vi "10_DiDt_OFF.vi"(0 "file path (IN)":path, 1 "ICE":dbl, 5 "Project #":string, 7 "Request #":string, 9 "TEST #":string, 11 "error in (no error)":errorcluster) -> (4 "file path (OUT)":path, 6 "Di/Dt (A/us)":dbl, 8 "DONE Di/Dt OFF":bool, 10 "OFF Region":waveform(dbl)[](graph) caption="DiDtOff (A/us)", 13 "Di (A)":dbl, 14 "Dt (ns)":dbl, 15 "error out":errorcluster)   [LabVIEW 2020]
uses:
  <vilib>/Waveform/WDTOps.llb/WDT Waveform Duration DBL.vi
  <vilib>/Waveform/WDTOps.llb/WDT Get Waveform Subset DBL.vi
  <vilib>/measure/mascope.llb/Transition Measurements 1 chan.vi
  <vilib>/measure/NI_MAPro.lvlib
panel:
  in  "Decision ?":bool
  out "Cursor b : Channel 1":dbl
  out "Cursor a : Channel 1":dbl
  in  "Cursor b : Channel 1 \nfall edge number":i32=1 min=1
  in  "Cursor b : Channel 1 \nfall edge tolerance":dbl=0.1
  in  "Cursor a : Channel 1 \nfall edge tolerance":dbl=0.1
  in  "Cursor a : Channel 1 \nfall edge number":i32=1 min=1
  out "Dt (us)":dbl
  out "50% Ice":dbl
  out "90% Ice":dbl
  out "measurement info (CH1 Cursor a)":T1 {"ref levels"."ref units" items=["absolute", "relative"]; "ref levels"."high ref level" format="%.2p"; "ref levels"."low ref level" format="%.2p"; "ref levels"."mid ref level" format="%.2p"; "end time" format="%.6e"; "start time" format="%.6e"}
  out "measurement info (CH1 Cursor b)":T1 {"ref levels"."ref units" items=["absolute", "relative"]; "ref levels"."high ref level" format="%.2p"; "ref levels"."low ref level" format="%.2p"; "ref levels"."mid ref level" format="%.2p"; "end time" format="%.6e"; "start time" format="%.6e"}
  in  "reference  levels (CH1 2nd Cursor)":T2={"high ref level"=90.0, "mid ref level"=50.0, "low ref level"=10.0, "ref units"=1} {"ref units" items=["absolute", "percent"]; "high ref level" format="%0.2f"; "low ref level" format="%0.2f"; "mid ref level" format="%0.2f"}
  in  "reference  levels (CH1 1st Cursor)":T2={"high ref level"=90.0, "mid ref level"=50.0, "low ref level"=10.0, "ref units"=1} {"ref units" items=["absolute", "percent"]; "high ref level" format="%0.2f"; "low ref level" format="%0.2f"; "mid ref level" format="%0.2f"}
  out "Waveform Graph":waveform(dbl)[](graph)
  # "From 90% to 50% of Nominal Current"
  # "Default = 1"
  # "Default = 1"
  # "Default = 0.1"
  # "Default = 0.1"
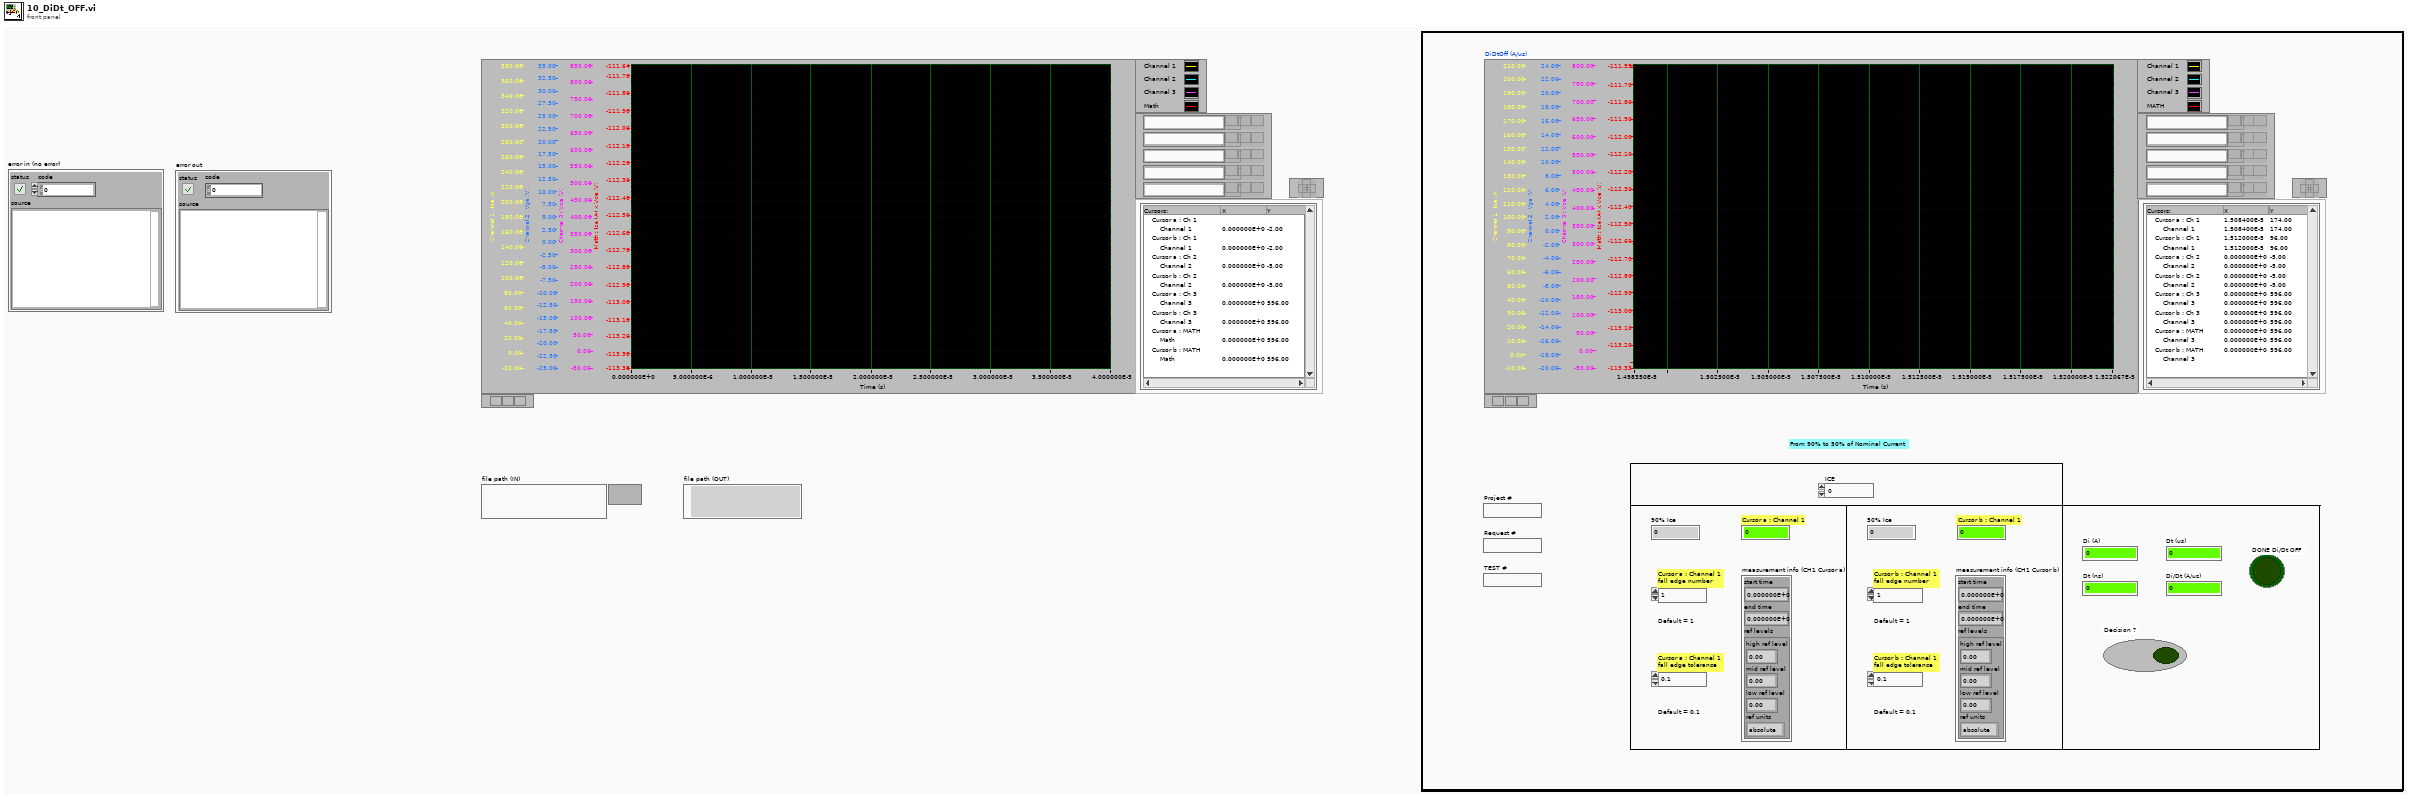
[diagram p1: front panel]
types:
  T1 = cluster{"start time":dbl, "end time":dbl, "ref levels":cluster{"high ref level":dbl, "mid ref level":dbl, "low ref level":dbl, "ref units":u16}}
  T2 = cluster{"high ref level":dbl, "mid ref level":dbl, "low ref level":dbl, "ref units":u16}
  T3 = enum32{"Invalid", "Standard", "Closed", "Hidden", "Minimized", "Maximized"}
  T4 = typedef "imagedata.ctl" = cluster{"image type":i32, "image depth":i32, "image":u8[], "mask":u8[], "colors":u32[], "Rectangle":cluster{"left":i16, "top":i16, "right":i16, "bottom":i16}}
diagram:
  w12 = 0.0 ("Di (A)")
  w13 = errorcluster {"status"=FALSE, "code"=0, "source"=""} ("error out")
  w11 = FALSE ("DONE Tdon")
  w14 = waveform(dbl)[] [] ("Waveform Graph")
  n1 = disable-structure shown="Disabled" {
    frame Disabled {
      n2 = control-ref of="This VI"() -> (w15:refnum<vi>)
      n3 = control-ref of="This VI"() -> (w16:refnum<vi>)
      n4 = invoke class="VI" method="FP.Close"(reference=w15) -> ()  [unwired: 2 in, 3 out]
      n5 = invoke class="VI" method="FP.Open"(reference=w16, "Activate"=TRUE ("Activate?"), "State"=T3."Maximized") -> (error in=w19:errorcluster, error out=w17:errorcluster)  [unwired: 1 in, 4 out]
      n6 = property class="VI"(reference=w16, error in=w17, "Front Panel.Closeable"=TRUE ("Front Panel Window:Closeable")) -> ()  [unwired: 2 out]
    }
    frame Enabled {
    }
  }
  n7 = local write "Cursor a : Channel 1 \nfall edge tolerance"(0.1 ("Cursor a : Channel 1 \nfall edge tolerance")) -> ()
  n8 = local write "Cursor a : Channel 1 \nfall edge number"(1 ("Cursor a : Channel 1 \nfall edge number")) -> ()
  n9 = local write "Cursor b : Channel 1 \nfall edge number"(1 ("Cursor b : Channel 1 \nfall edge number")) -> ()
  n10 = local write "Cursor b : Channel 1 \nfall edge tolerance"(0.1 ("Cursor b : Channel 1 \nfall edge tolerance")) -> ()
  n11 = local write "Cursor a : Channel 1"(w12) -> ()
  n12 = local write "Cursor b : Channel 1"(w12) -> ()
  n13 = local write "Di (A)"(w12) -> ()
  n14 = local write "Dt (ns)"(w12) -> ()
  n15 = local write "Dt (us)"(w12) -> ()
  n16 = local write "Di/Dt (A/us)"(w12) -> ()
  n17 = local write "error out"(w13) -> ()
  n18 = local write "error in (no error)"(w13) -> ()
  n19 = local write "DONE Di/Dt OFF"(w11) -> ()
  n20 = local write "Waveform Graph"(w14) -> ()
  n21 = local write "OFF Region"(w14) -> ()
  n22 = local write "Decision ?"(w11) -> ()
  n23 = flat-sequence {
    tunnel: [w22] -> w6
    tunnel: ["file path (IN)"] -> w5
    tunnel: [w33] -> w10
    tunnel: [w32] -> w8
    tunnel: w6 -> [w31]
    tunnel: w5 -> [w30]
    tunnel: w10 -> [w265]
    tunnel: [w264] -> w9
    tunnel: w8 -> [w264]
    tunnel: [w263] -> w7
    tunnel: w9 -> [w279]
    tunnel: w7 -> [w278]
    frame #0 {
      n24 = control-ref of="This VI"() -> (w27:refnum<vi>)
      n25 = invoke class="VI" method="FP.Open"(reference=w27, error in="error in (no error)", "Activate"=TRUE ("Activate?"), "State"=T3."Maximized") -> (error out=w28:errorcluster)  [unwired: 1 in, 4 out]
      n26 = property class="VI"(reference=w27, error in=w28, "Front Panel.Closeable"=TRUE ("Front Panel Window:Closeable")) -> (error out=w22:errorcluster)  [unwired: 1 out]
    }
    frame #1 {
      n27 = while {
        tunnel: [w37] -> w32
        shift-right: [w38] -> w33
        shift-left: w31 -> [w36]
        tunnel: w30 -> [w35]
        stop <- w40 stop-if-true
        n28 = flat-sequence {
          tunnel: [w71] -> w59
          tunnel: w36 -> [w71]
          tunnel: w35 -> [w66]
          tunnel: [w66] -> w34
          tunnel: w59 -> [w164]
          tunnel: [w87] -> w58
          tunnel: [w86] -> w57
          tunnel: [w76] -> w56
          tunnel: w34 -> [w158]
          tunnel: w58 -> [w193]
          tunnel: w57 -> [w207]
          tunnel: [w187] -> w55
          tunnel: w56 -> [w200]
          tunnel: [w200] -> w54
          tunnel: [w178] -> w53
          tunnel: [w177] -> w52
          tunnel: [w186] -> w51
          tunnel: [w185] -> w50
          tunnel: w55 -> [w234]
          tunnel: [w235] -> w49
          tunnel: w54 -> [w238]
          tunnel: [w238] -> w48
          tunnel: w53 -> [w237]
          tunnel: [w237] -> w47
          tunnel: w52 -> [w236]
          tunnel: [w236] -> w46
          tunnel: w51 -> [w228]
          tunnel: [w228] -> w45
          tunnel: w50 -> [w229]
          tunnel: [w229] -> w44
          tunnel: w49 -> [w239]
          tunnel: w48 -> [w252]
          tunnel: [w252] -> w43
          tunnel: w47 -> [w246]
          tunnel: w46 -> [w247]
          tunnel: w45 -> [w245]
          tunnel: w44 -> [w244]
          tunnel: [w239] -> w42
          tunnel: w43 -> [w257]
          tunnel: w42 -> [w259]
          tunnel: [w258] -> w41
          tunnel: [w257] -> w37
          frame #0 {
            w69 = 0.0 ("Di (A)")
            w70 = FALSE ("DONE Tdon")
            w68 = waveform(dbl)[] [] ("Waveform Graph")
            n29 = Wait (ms)(milliseconds to wait=u32 200) -> ()  [unwired: 1 out]
            n30 = local write "Cursor a : Channel 1"(w69) -> ()
            n31 = local write "Cursor b : Channel 1"(w69) -> ()
            n32 = local write "Di/Dt (A/us)"(w69) -> ()
            n33 = local write "Dt (us)"(w69) -> ()
            n34 = local write "Di (A)"(w69) -> ()
            n35 = local write "Dt (ns)"(w69) -> ()
            n36 = local write "DONE Di/Dt OFF"(w70) -> ()
            n37 = local write "Waveform Graph"(w68) -> ()
            n38 = local write "OFF Region"(w68) -> ()
            n39 = local write "Decision ?"(w70) -> ()
          }
          frame #1 {
            w72 = 0.0 ("start samples/time")
            w139 = u16 1 items=["Samples", "Relative Time"] ("start/duration format")
            w150 = u16 1 items=["Samples", "Relative Time"] ("start/duration format")
            w151 = u16 1 items=["Samples", "Relative Time"] ("start/duration format")
            # "Channel 1"
            # "Channel 3"
            # "Channel 2"
            # "dt"
            # "Ch2"
            # "Ch1"
            n40 = call "3_ReadDatatoWaveform.vi"("error in (no error)"=w164, "file path (IN)"=w158) -> ("error out"=w132:errorcluster, "Waveform Graph"=→"Waveform Graph":waveform(dbl)[], "file path (OUT)"=w76:path, "dt"=w159:dbl, "Ch 2 Data"=w156:dbl[], "Ch 3 Data"=w160:dbl[], "Ch 1 Data"=w157:dbl[])  [unwired: 3 in]
            n41 = To Time Stamp(1:0.0 ("number")) -> (0:w161:timestamp)
            n42 = disable-structure shown="Enabled" {
              disable-tunnel: w161 -> [w168 _]
              disable-tunnel: w159 -> [w167 _]
              disable-tunnel: w157 -> [w166 _]
              disable-tunnel: [w165 _] -> w138
              frame Enabled {
                # "Channel 1"
                n43 = Bundle By Name("Y"=w166, "dt"=w167, "t0"=w168) -> (w165:waveform(dbl))  [unwired: 1 in]
              }
              frame Disabled {
              }
            }
            n44 = disable-structure shown="Enabled" {
              disable-tunnel: w161 -> [w172 _]
              disable-tunnel: w159 -> [w171 _]
              disable-tunnel: w156 -> [w170 _]
              disable-tunnel: [w169 _] -> w137
              frame Enabled {
                # "Channel 2"
                n45 = Bundle By Name("Y"=w170, "dt"=w171, "t0"=w172) -> (w169:waveform(dbl))  [unwired: 1 in]
              }
              frame Disabled {
              }
            }
            n46 = disable-structure shown="Enabled" {
              disable-tunnel: w161 -> [w176 _]
              disable-tunnel: w159 -> [w175 _]
              disable-tunnel: w160 -> [w174 _]
              disable-tunnel: [w173 _] -> w136
              frame Enabled {
                # "Channel 3"
                n47 = Bundle By Name("Y"=w174, "dt"=w175, "t0"=w176) -> (w173:waveform(dbl))  [unwired: 1 in]
              }
              frame Disabled {
              }
            }
            n48 = call-poly <vilib>:"Waveform Duration.vi"("error in (no error)"=w132, "waveform in"=w136) -> ("error out"=w144:errorcluster, "duration"=w141:dbl, "waveform out"=w143:waveform(dbl))  [unwired: 7 in]
            n49 = call-poly <vilib>:"Waveform Duration.vi"("error in (no error)"=w132, "waveform in"=w137) -> ("error out"=w145:errorcluster, "duration"=w148:dbl, "waveform out"=w146:waveform(dbl))  [unwired: 7 in]
            n50 = call-poly <vilib>:"Waveform Duration.vi"("error in (no error)"=w132, "waveform in"=w138) -> ("error out"=w155:errorcluster, "duration"=w152:dbl, "waveform out"=w154:waveform(dbl))  [unwired: 7 in]
            n51 = Divide(x=w141, y=2.0) -> (x/y=w140:dbl)
            n52 = Divide(x=w148, y=2.0) -> (x/y=w149:dbl)
            n53 = Divide(x=w152, y=2.0) -> (x/y=w133:dbl)
            n54 = call-poly <vilib>:"Get Waveform Subset.vi"("start/duration format"=w139, "error in (no error)"=w144, "duration"=w140, "start samples/time"=w72, "waveform in"=w143) -> ("error out"=w129:errorcluster, "waveform out"=w135:waveform(dbl))  [unwired: 1 in, 2 out]
            n55 = call-poly <vilib>:"Get Waveform Subset.vi"("start/duration format"=w150, "error in (no error)"=w145, "duration"=w149, "start samples/time"=w72, "waveform in"=w146) -> ("error out"=w130:errorcluster, "waveform out"=w88:waveform(dbl))  [unwired: 1 in, 2 out]
            n56 = call-poly <vilib>:"Get Waveform Subset.vi"("start/duration format"=w151, "error in (no error)"=w155, "duration"=w133, "start samples/time"=w72, "waveform in"=w154) -> ("error out"=w131:errorcluster, "waveform out"=w87:waveform(dbl))  [unwired: 1 in, 2 out]
            n57 = Build Array(w87, w88, w135) -> (→"OFF Region":waveform(dbl)[])
            n58 = Merge Errors(w131, w130, w129) -> (w84:errorcluster)
            n59 = property on="OFF Region" class="WFGraph (strict)"(error in=w84) -> (error out=w83:errorcluster, "Width"=w82:u32)  [unwired: 1 in, 1 out]
            n60 = property on="OFF Region" class="WFGraph (strict)"(error in=w83, "Caption.Justify"=enum16{"Left", "Center", "Right"}."Left" ("Caption.Justification"), "Caption.Width"=w82, "Caption.FontBold"=TRUE ("Caption.Font:Bold"), "Caption.FontColor"=u32 16860 ("Caption.Font:Color"), "Caption.FontSize"=u32 24 ("Caption.Font:Size"), "Caption.Text"="DiDtOff (A/us)") -> (error out=w78:errorcluster)  [unwired: 1 in, 1 out]
            n61 = property on="OFF Region" class="WFGraph (strict)"(error in=w78, "XScale.Offset"=w72) -> (error out=w112:errorcluster)  [unwired: 1 in, 1 out]
            n62 = property on="OFF Region" class="WFGraph (strict)"(error in=w112, "Active Cursor"=u32 0, "Cursor.Cursor X"=0.0 ("Cursor.Cursor Position:Cursor X"), "Cursor.Cursor Y"=0.0 ("Cursor.Cursor Position:Cursor Y"), "Cursor.Visible"=FALSE) -> (error out=w111:errorcluster)  [unwired: 1 in, 1 out]
            n63 = property on="OFF Region" class="WFGraph (strict)"(error in=w111, "Active Cursor"=u32 1, "Cursor.Cursor X"=0.0 ("Cursor.Cursor Position:Cursor X"), "Cursor.Cursor Y"=0.0 ("Cursor.Cursor Position:Cursor Y"), "Cursor.Visible"=FALSE) -> (error out=w110:errorcluster)  [unwired: 1 in, 1 out]
            n64 = property on="OFF Region" class="WFGraph (strict)"(error in=w110, "Active Cursor"=u32 2, "Cursor.Cursor X"=0.0 ("Cursor.Cursor Position:Cursor X"), "Cursor.Cursor Y"=0.0 ("Cursor.Cursor Position:Cursor Y"), "Cursor.Visible"=FALSE) -> (error out=w109:errorcluster)  [unwired: 1 in, 1 out]
            n65 = property on="OFF Region" class="WFGraph (strict)"(error in=w109, "Active Cursor"=u32 3, "Cursor.Cursor X"=0.0 ("Cursor.Cursor Position:Cursor X"), "Cursor.Cursor Y"=0.0 ("Cursor.Cursor Position:Cursor Y"), "Cursor.Visible"=FALSE) -> (error out=w92:errorcluster)  [unwired: 1 in, 1 out]
            n66 = property on="OFF Region" class="WFGraph (strict)"(error in=w92, "Active Cursor"=u32 4, "Cursor.Cursor X"=0.0 ("Cursor.Cursor Position:Cursor X"), "Cursor.Cursor Y"=0.0 ("Cursor.Cursor Position:Cursor Y"), "Cursor.Visible"=FALSE) -> (error out=w91:errorcluster)  [unwired: 1 in, 1 out]
            n67 = property on="OFF Region" class="WFGraph (strict)"(error in=w91, "Active Cursor"=u32 5, "Cursor.Cursor X"=0.0 ("Cursor.Cursor Position:Cursor X"), "Cursor.Cursor Y"=0.0 ("Cursor.Cursor Position:Cursor Y"), "Cursor.Visible"=FALSE) -> (error out=w90:errorcluster)  [unwired: 1 in, 1 out]
            n68 = property on="OFF Region" class="WFGraph (strict)"(error in=w90, "Active Cursor"=u32 6, "Cursor.Cursor X"=0.0 ("Cursor.Cursor Position:Cursor X"), "Cursor.Cursor Y"=0.0 ("Cursor.Cursor Position:Cursor Y"), "Cursor.Visible"=FALSE) -> (error out=w89:errorcluster)  [unwired: 1 in, 1 out]
            n69 = property on="OFF Region" class="WFGraph (strict)"(error in=w89, "Active Cursor"=u32 7, "Cursor.Cursor X"=0.0 ("Cursor.Cursor Position:Cursor X"), "Cursor.Cursor Y"=0.0 ("Cursor.Cursor Position:Cursor Y"), "Cursor.Visible"=FALSE) -> (error out=w86:errorcluster)  [unwired: 1 in, 1 out]
            n70 = call <vilib>:"Beep.vi"("use system alert? (T)"=FALSE, "duration (msec)"=u32 200, "frequency (Hz)"=u32 2000) -> ()  [unwired: 9 in]
          }
          frame #2 {
            w220 = u16 0 items=["falling", "rising"] ("polarity (rising)")
            w221 = u16 0 items=["falling", "rising"] ("polarity (rising)")
            # "XPOS"
            # "YPOS"
            # "Cursor a : Channel 1"
            # "Cursor b : Channel 1"
            # "Cursor b : Channel 1"
            # "Cursor a : Channel 1"
            # "Cursor b : Channel 1"
            # "Cursor a : Channel 1"
            # "Cursor b : Channel 1"
            # "Cursor a : Channel 1"
            # "End Time 1st Cursor"
            # "End Time 2nd Cursor"
            # "1st PARAMETER : 90% Ice"
            # "Channel 1"
            # "2nd PARAMETER : 50% Ice"
            # "Channel 1"
            n71 = Divide(x=90.0, y=100.0) -> (x/y=w227:dbl)
            n72 = Multiply(x=w227, y="ICE") -> (x*y=w195:dbl)
            "90% Ice" <- w195
            n73 = Add(x=w195, y="Cursor a : Channel 1 \nfall edge tolerance") -> (x+y=w213:dbl)
            n74 = Subtract(x=w195, y="Cursor a : Channel 1 \nfall edge tolerance") -> (x-y=w212:dbl)
            n75 = Bundle By Name(cluster="reference  levels (CH1 1st Cursor)", "high ref level"=w213, "mid ref level"=w195, "low ref level"=w212, "ref units"=u16 0) -> (w209:T2)
            n76 = call-poly <vilib>:"Transition Measurements.vi"("edge number (1)"="Cursor a : Channel 1 \nfall edge number", "error in (no error)"=w207, "reference levels"=w209, "polarity (rising)"=w221, "signal in"=w193) -> ("error out"=w204:errorcluster, "measurement info"=w208:T1)  [unwired: 1 in, 4 out]
            "measurement info (CH1 Cursor a)" <- w208
            n77 = Unbundle By Name(w208) -> ("end time"=w185:dbl)
            n78 = property on="OFF Region" class="WFGraph (strict)"(error in=w204, "Active Cursor"=u32 0, "Cursor.Cursor X"=w185, "Cursor.Visible"=TRUE, "Cursor.Cursor Name Visible"=TRUE) -> (error out=w192:errorcluster)  [unwired: 1 in, 1 out]
            n79 = property on="OFF Region" class="WFGraph (strict)"(error in=w192, "Active Cursor"=u32 0) -> (error out=w190:errorcluster, "Cursor.Cursor Y"=w178:dbl)  [unwired: 1 in, 1 out]
            "Cursor a : Channel 1" <- w178
            n80 = Divide(x=50.0, y=100.0) -> (x/y=w224:dbl)
            n81 = Multiply(x=w224, y="ICE") -> (x*y=w196:dbl)
            "50% Ice" <- w196
            n82 = Add(x=w196, y="Cursor b : Channel 1 \nfall edge tolerance") -> (x+y=w219:dbl)
            n83 = Subtract(x=w196, y="Cursor b : Channel 1 \nfall edge tolerance") -> (x-y=w218:dbl)
            n84 = Bundle By Name(cluster="reference  levels (CH1 2nd Cursor)", "high ref level"=w219, "mid ref level"=w196, "low ref level"=w218, "ref units"=u16 0) -> (w215:T2)
            n85 = call-poly <vilib>:"Transition Measurements.vi"("edge number (1)"="Cursor b : Channel 1 \nfall edge number", "error in (no error)"=w190, "reference levels"=w215, "polarity (rising)"=w220, "signal in"=w193) -> ("error out"=w201:errorcluster, "measurement info"=w214:T1)  [unwired: 1 in, 4 out]
            "measurement info (CH1 Cursor b)" <- w214
            n86 = Unbundle By Name(w214) -> ("end time"=w186:dbl)
            n87 = property on="OFF Region" class="WFGraph (strict)"(error in=w201, "Active Cursor"=u32 1, "Cursor.Cursor X"=w186, "Cursor.Visible"=TRUE, "Cursor.Cursor Name Visible"=TRUE) -> (error out=w188:errorcluster)  [unwired: 1 in, 1 out]
            n88 = call <vilib>:"Beep.vi"("use system alert? (T)"=FALSE, "duration (msec)"=u32 200, "frequency (Hz)"=u32 2000) -> ()  [unwired: 9 in]
            n89 = property on="OFF Region" class="WFGraph (strict)"(error in=w188, "Active Cursor"=u32 1) -> (error out=w187:errorcluster, "Cursor.Cursor Y"=w177:dbl)  [unwired: 1 in, 1 out]
            "Cursor b : Channel 1" <- w177
          }
          frame #3 {
            # "2nd Cursor"
            # "1st Cursor"
            n90 = Subtract(x=w229, y=1e-07) -> (x-y=w230:dbl)
            n91 = Add(x=w228, y=1e-07) -> (x+y=w231:dbl)
            n92 = property on="OFF Region" class="WFGraph (strict)"(error in=w234, "XScale.Minimum"=w230, "XScale.Maximum"=w231) -> (error out=w235:errorcluster)  [unwired: 1 in, 1 out]
          }
          frame #4 {
            # "us"
            # "ns"
            n93 = Subtract(x=w247, y=w246) -> (x-y=w242:dbl)
            n94 = Subtract(x=w245, y=w244) -> (x-y=w243:dbl)
            n95 = Absolute Value(x=w242) -> (abs(x)=w241:dbl)
            "Di (A)" <- w241
            n96 = Absolute Value(x=w243) -> (abs(x)=w240:dbl)
            n97 = Multiply(x=w240, y=1000000000.0) -> (x*y=→"Dt (ns)":dbl)
            n98 = Multiply(x=w240, y=1000000.0) -> (x*y=w249:dbl)
            "Dt (us)" <- w249
            n99 = Divide(x=w241, y=w249) -> (x/y=→"Di/Dt (A/us)":dbl)
            n100 = call <vilib>:"Beep.vi"("use system alert? (T)"=FALSE, "duration (msec)"=u32 200, "frequency (Hz)"=u32 2000) -> ()  [unwired: 9 in]
          }
          frame #5 {
            n101 = while {
              shift-right: [w260] -> w258
              shift-left: w259 -> [w260]
              stop <- "Decision ?" stop-if-true
              n102 = Wait (ms)(milliseconds to wait=u32 100) -> ()  [unwired: 1 out]
            }
          }
        }
        n103 = while {
          tunnel: [w61] -> w40
          shift-right: [w64] -> w38
          shift-left: w41 -> [w65]
          stop <- w63 stop-if-true
          n104 = Wait (ms)(milliseconds to wait=u32 100) -> ()  [unwired: 1 out]
          n105 = call "Display Message to User"("error in (no error)"=w65) -> ("error out"=w64:errorcluster, "NO"=w61:bool)  [unwired: 9 in]
          n106 = Or(x=w61, y=TRUE) -> (x .or. y?=w63:bool)
        }
        n107 = Wait (ms)(milliseconds to wait=u32 100) -> ()  [unwired: 1 out]
      }
    }
    frame #2 {
      w268 = "_"
      n108 = invoke on="OFF Region" class="WFGraph (strict)" method="Get Image"(error in=w265) -> (error out=w271:errorcluster, "image data"=w274:T4)  [unwired: 5 in, 4 out]
      n109 = Concatenate Strings("C:\\Inductive_Switching_Project\\IndSw_Image\\" ("string"), "Project #", w268, "Request #", w268, "TEST #", w268, "DiDtOff" ("string"), ".png" ("string")) -> (w275:string)
      n110 = String To Path(string=w275) -> (path=w273:path)
      n111 = call <vilib>:"Write PNG File.vi"("error in (no error)"=w271, "image data"=w274, "path to PNG file"=w273) -> ("error out"=w263:errorcluster)  [unwired: 7 in, 1 out]
      "DONE Di/Dt OFF" <- TRUE ("DONE Di/Dt ON")
    }
    frame #3 {
      n112 = disable-structure shown="Enabled" {
        disable-tunnel: w278 -> [w280 _]
        frame Enabled {
          n113 = control-ref of="This VI"() -> (w281:refnum<vi>)
          n114 = invoke class="VI" method="FP.Close"(reference=w281, error in=w280) -> ()  [unwired: 1 in, 3 out]
        }
        frame Disabled {
        }
      }
      "error out" <- w278
      "file path (OUT)" <- w279
    }
  }
